vi "manual_piezo_and_z.vi"(1 "Stop Button":bool) -> ()   [LabVIEW 2012]
uses:
  <vilib>/Utility/error.llb/DialogType.ctl
  <vilib>/DAQmx/write.llb/DAQmx Write (Analog DBL 1Chan 1Samp).vi
  <vilib>/DAQmx/create/channels.llb/DAQmx Create Channel (AO-Voltage-Basic).vi
  <vilib>/DAQmx/miscellaneous.llb/DAQmx Fill In Error Info.vi
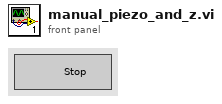
[diagram p1: front panel]
types:
  T1 = typedef "DialogType.ctl" = u16
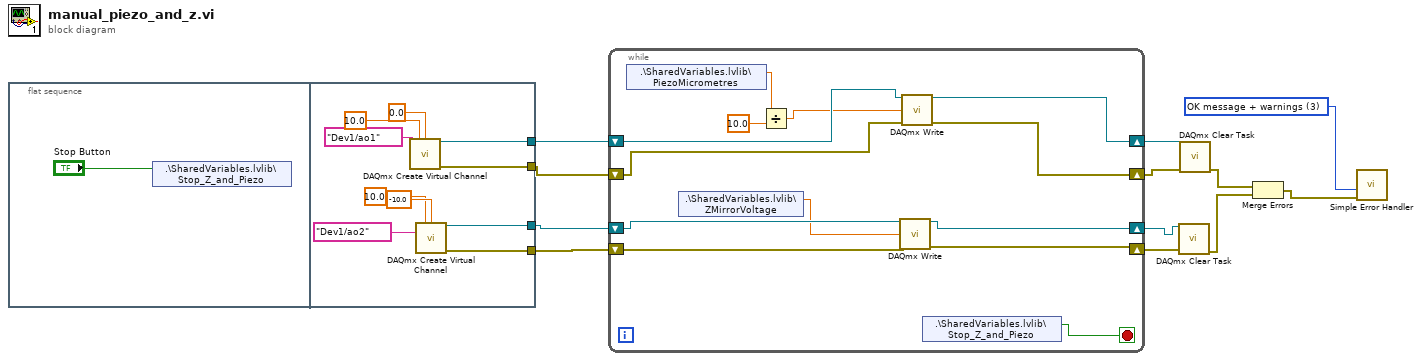
[diagram p0: block diagram]
diagram:
  w4 = T1 3 items=["no dialog", "OK message", "continue or stop message", "OK message + warnings", "continue/stop + warnings"] ("type of dialog (OK msg:1)")
  n1 = flat-sequence {
    tunnel: [w19] -> w12
    tunnel: [w18] -> w11
    tunnel: [w17] -> w8
    tunnel: [w16] -> w7
    frame #0 {
      n2 = shared-variable ".\\SharedVariables.lvlib\\Stop_Z_and_Piezo"("Stop Button") -> ()  [unwired: 1 in, 1 out]
    }
    frame #1 {
      n3 = call-poly <vilib>:"DAQmx Create Virtual Channel.vi"("maximum value"=10.0, "minimum value"=0.0, "physical channels"=tag "Dev1/ao1") -> ("task out"=w19:refnum<k21>, "error out"=w18:errorcluster)  [unwired: 11 in]
      n4 = call-poly <vilib>:"DAQmx Create Virtual Channel.vi"("maximum value"=10.0, "minimum value"=-10.0, "physical channels"=tag "Dev1/ao2") -> ("task out"=w17:refnum<k21>, "error out"=w16:errorcluster)  [unwired: 11 in]
    }
  }
  n5 = while {
    shift-right: [w35] -> w10
    shift-left: w12 -> [w36]
    shift-right: [w33] -> w9
    shift-left: w11 -> [w34]
    shift-right: [w30] -> w6
    shift-left: w8 -> [w32]
    shift-right: [w29] -> w5
    shift-left: w7 -> [w31]
    stop <- w28 stop-if-true
    n6 = shared-variable ".\\SharedVariables.lvlib\\PiezoMicrometres"() -> (w26:dbl)  [unwired: 1 in, 1 out]
    n7 = shared-variable ".\\SharedVariables.lvlib\\ZMirrorVoltage"() -> (w24:dbl)  [unwired: 1 in, 1 out]
    n8 = Divide(x=w26, y=10.0) -> (x/y=w25:dbl)
    n9 = call-poly <vilib>:"DAQmx Write.vi"("task/channels in"=w32, "data"=w24, "error in"=w31) -> ("task out"=w30:refnum<k21>, "error out"=w29:errorcluster)  [unwired: 10 in, 1 out]
    n10 = call-poly <vilib>:"DAQmx Write.vi"("task/channels in"=w36, "data"=w25, "error in"=w34) -> ("task out"=w35:refnum<k21>, "error out"=w33:errorcluster)  [unwired: 10 in, 1 out]
    n11 = shared-variable ".\\SharedVariables.lvlib\\Stop_Z_and_Piezo"() -> (w28:bool)  [unwired: 1 in, 1 out]
  }
  n12 = call <vilib>:"DAQmx Clear Task.vi"("task in"=w6, "error in"=w5) -> ("error out"=w2:errorcluster)  [unwired: 13 in]
  n13 = call <vilib>:"DAQmx Clear Task.vi"("task in"=w10, "error in"=w9) -> ("error out"=w3:errorcluster)  [unwired: 13 in]
  n14 = Merge Errors(w3, w2) -> (w1:errorcluster)
  n15 = call <vilib>:"Simple Error Handler.vi"("type of dialog (OK msg:1)"=w4, "error in (no error)"=w1) -> ()  [unwired: 3 in, 5 out]
